vi "Replace NaN in Measurements.vi"(0 "Measurements":dbl[](array[numeric])) -> (4 "Measurements":dbl[](array[numeric]))   [LabVIEW 2024, in "devicePowerSequencerCoreLogic.lvlib"]
uses:
  devicePowerSequencerCoreLogic.lvlib
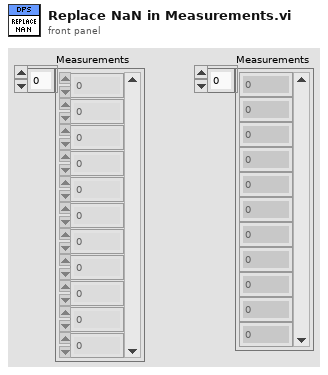
[diagram p1: front panel]
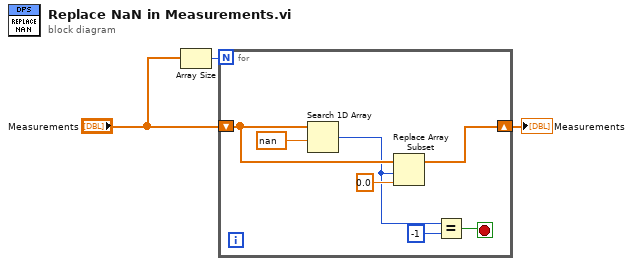
[diagram p0: block diagram]
diagram:
  n1 = Array Size(array="Measurements") -> (size(s)=w2:i32)
  n2 = for {
    N: w2 -> [_]
    shift-right: [w7] -> w3
    shift-left: "Measurements" -> [w8]
    stop <- w6 stop-if-true
    n3 = Search 1D Array(1D array=w8, element=nan) -> (index of element=w5:i32)  [unwired: 1 in]
    n4 = Replace Array Subset(array=w8, new element=0.0 ("new element/subarray"), index=w5) -> (w7:dbl[])
    n5 = Equal?(x=w5, y=-1) -> (x = y?=w6:bool)
  }
  "Measurements" <- w3
